vi "LogWatchDogFailure.vi"(8 "error in (no error)":errorcluster, 10 "Elapsed":bool[](array[boolean])) -> (0 "error out":errorcluster)   [LabVIEW 2018]
panel:
  out "Watchdog Failure String":string
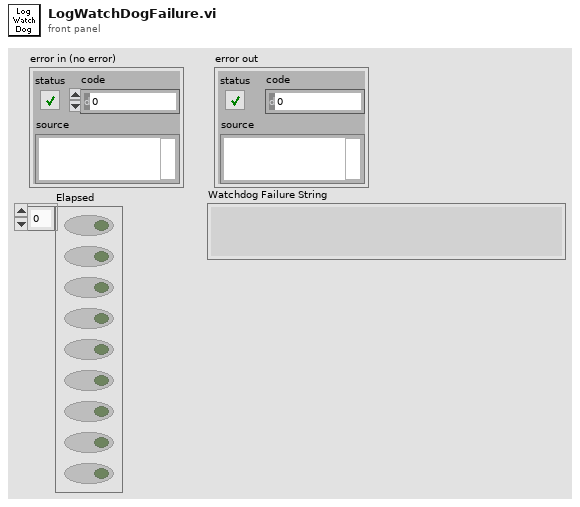
[diagram p1: front panel]
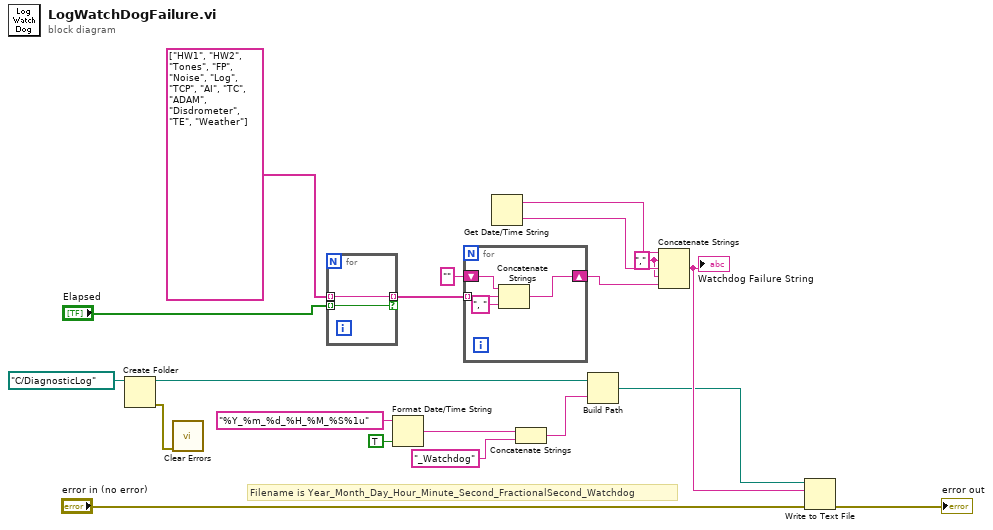
[diagram p0: block diagram]
diagram:
  w6 = "," ("string")
  # "Filename is Year_Month_Day_Hour_Minute_Second_FractionalSecond_Watchdog"
  n1 = Create Folder(path (use dialog)=path "C:/DiagnosticLog" ("file path (use dialog)")) -> (created path=w9:path, error out=w8:errorcluster)  [unwired: 2 in, 1 out]
  n2 = call <vilib>:"Clear Errors.vi"("error in (no error)"=w8) -> ()  [unwired: 5 in, 2 out]
  n3 = for {
    tunnel: "Elapsed" -> [w21] mode=indexing
    tunnel: [w22] -> w16 mode=indexing if=w21
    tunnel: string[] ["HW1", "HW2", "Tones", "FP", "Noise", "Log", "TCP", "AI", "TC", "ADAM", "Disdrometer", "TE", "Weather"] -> [w22] mode=indexing
  }
  n4 = Format Date/Time String(time format string (%c)="%Y_%m_%d_%H_%M_%S%1u", UTC format=TRUE) -> (date/time string=w3:string)  [unwired: 1 in]
  n5 = for {
    tunnel: w16 -> [w26] mode=indexing
    shift-right: [w25] -> w14
    shift-left: "" -> [w24]
    n6 = Concatenate Strings(w24, w26, ", " ("string")) -> (w25:string)
  }
  n7 = Get Date/Time String() -> (date string=w13:string, time string=w12:string)  [unwired: 3 in]
  n8 = Concatenate Strings(w3, "_Watchdog" ("name or relative path")) -> (w1:string)
  n9 = Build Path(base path=w9, name or relative path=w1) -> (appended path=w7:path)
  n10 = Concatenate Strings(w13, w6, w12, w6, w14) -> (w11:string)
  "Watchdog Failure String" <- w11
  n11 = Write to Text File(file (use dialog)=w7, text=w11, error in="error in (no error)") -> (error out=→"error out":errorcluster)  [unwired: 1 in, 2 out]
